vi "SNMP Type to String.vi"(1 "Data":u8[](array[numeric]) format="%.0x", 2 "Type":u8) -> (0 "TypeAsString":string)   [LabVIEW 2017]
doc: "This VI is used to convert the numeric data to a string representation. The input to this VI is the raw byte array containing the data as read from the PDU. The data will be converted according to the specified data type into an ASCII string."
panel:
  out "OctetStringAsBinary":bool
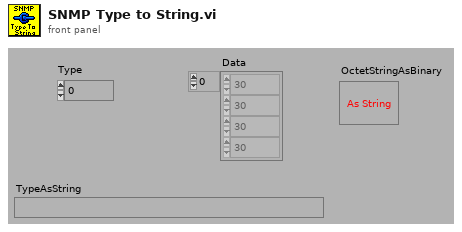
[diagram p1: front panel]
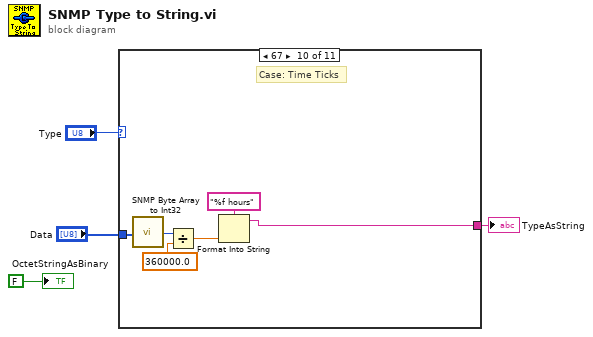
[diagram p0: block diagram]
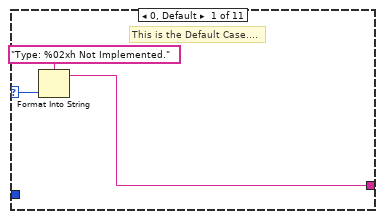
[diagram p2: hidden frame]
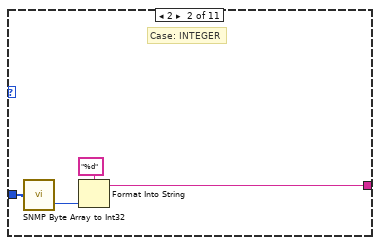
[diagram p3: hidden frame]
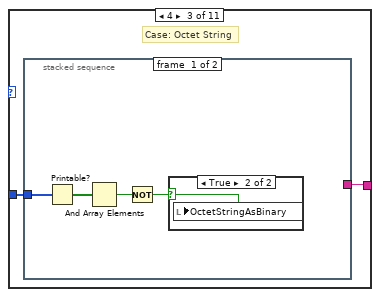
[diagram p4: hidden frame]
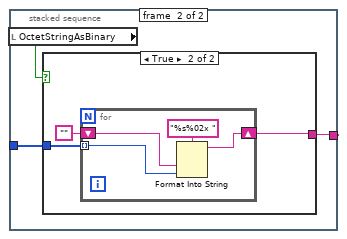
[diagram p6: hidden frame]
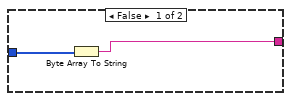
[diagram p7: hidden frame]
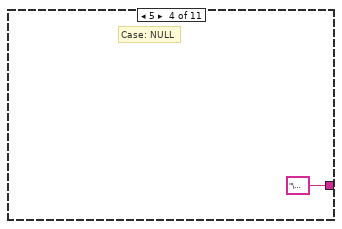
[diagram p8: hidden frame]
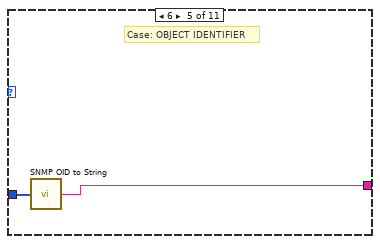
[diagram p9: hidden frame]
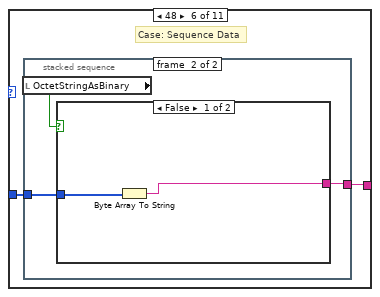
[diagram p10: hidden frame]
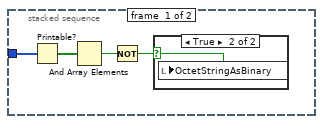
[diagram p11: hidden frame]
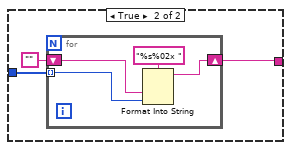
[diagram p13: hidden frame]
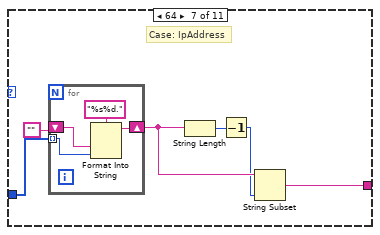
[diagram p14: hidden frame]
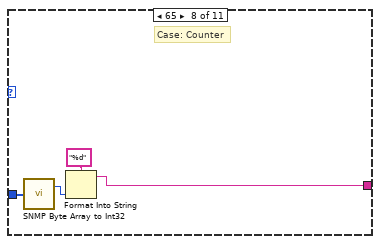
[diagram p15: hidden frame]
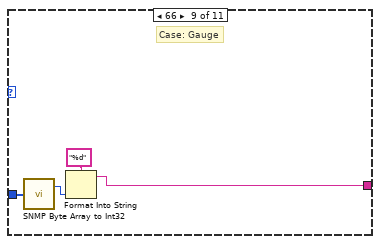
[diagram p16: hidden frame]
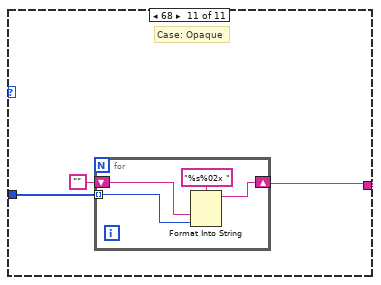
[diagram p17: hidden frame]
diagram:
  n1 = case shown="67" "Type" {
    selector: "Type" -> [w6 _ _ _ _ _ _ _ _ _ _]
    tunnel: "Data" -> [_ w10 w13 _ w33 w35 w57 w65 w68 w72 w79]
    tunnel: [w5 w9 w12 "\u0000" w32 w34 w53 w64 w67 w73 w78] -> w2
    frame 0, Default {
      # "This is the Default Case...."
      n2 = Format Into String(format string="Type: %02xh Not Implemented." ("OID String"), w6) -> (resulting string=w5:string)  [unwired: 2 in, 1 out]
    }
    frame 2 {
      # "Case: INTEGER"
      n3 = call "SNMP Byte Array to Int32.vi"("DataArray"=w10) -> ("Signed Value"=w8:i32)  [unwired: 1 out]
      n4 = Format Into String(format string="%d", w8) -> (resulting string=w9:string)  [unwired: 2 in, 1 out]
    }
    frame 4 {
      # "Case: Octet String"
      n5 = stacked-sequence {
        tunnel: w13 -> [w17 w20]
        tunnel: [_ w19] -> w12
        frame #0 {
          n6 = Printable?(1:w17) -> (0:w16:bool[])
          n7 = And Array Elements(Boolean array=w16) -> (logical AND=w15:bool)
          n8 = Not(x=w15) -> (.not. x?=w14:bool)
          n9 = case shown="True" w14 {
            selector: w14 -> [_ w18]
            frame False {
            }
            frame True {
              n10 = local write "OctetStringAsBinary"(w18) -> ()
            }
          }
        }
        frame #1 {
          n11 = local read "OctetStringAsBinary"() -> (w21:bool)
          n12 = case shown="True" w21 {
            tunnel: w20 -> [w23 w26]
            tunnel: [w22 w25] -> w19
            frame False {
              n13 = Byte Array To String(unsigned byte array=w23) -> (string=w22:string)
            }
            frame True {
              n14 = for {
                tunnel: w26 -> [w29] mode=indexing
                shift-right: [w27] -> w25
                shift-left: "" -> [w28]
                n15 = Format Into String(format string="%s%02x ", w28, w29) -> (resulting string=w27:string)  [unwired: 2 in, 1 out]
              }
            }
          }
        }
      }
    }
    frame 5 {
      # "Case: NULL"
    }
    frame 6 {
      # "Case: OBJECT IDENTIFIER"
      n16 = call "SNMP OID to String.VI"("OID"=w33) -> ("OID String"=w32:string)
    }
    frame 48 {
      # "Case: Sequence Data"
      n17 = stacked-sequence {
        tunnel: w35 -> [w39 w42]
        tunnel: [_ w41] -> w34
        frame #0 {
          n18 = Printable?(1:w39) -> (0:w38:bool[])
          n19 = And Array Elements(Boolean array=w38) -> (logical AND=w37:bool)
          n20 = Not(x=w37) -> (.not. x?=w36:bool)
          n21 = case shown="True" w36 {
            selector: w36 -> [_ w40]
            frame False {
            }
            frame True {
              n22 = local write "OctetStringAsBinary"(w40) -> ()
            }
          }
        }
        frame #1 {
          n23 = local read "OctetStringAsBinary"() -> (w43:bool)
          n24 = case shown="False" w43 {
            tunnel: w42 -> [w45 w48]
            tunnel: [w44 w47] -> w41
            frame False {
              n25 = Byte Array To String(unsigned byte array=w45) -> (string=w44:string)
            }
            frame True {
              n26 = for {
                tunnel: w48 -> [w51] mode=indexing
                shift-right: [w49] -> w47
                shift-left: "" -> [w50]
                n27 = Format Into String(format string="%s%02x ", w50, w51) -> (resulting string=w49:string)  [unwired: 2 in, 1 out]
              }
            }
          }
        }
      }
    }
    frame 64 {
      # "Case: IpAddress"
      n28 = for {
        tunnel: w57 -> [w61] mode=indexing
        shift-right: [w59] -> w56
        shift-left: "" -> [w60]
        n29 = Format Into String(format string="%s%d.", w60, w61) -> (resulting string=w59:string)  [unwired: 2 in, 1 out]
      }
      n30 = String Length(string=w56) -> (length=w55:i32)
      n31 = Decrement(x=w55) -> (x-1=w54:i32)
      n32 = String Subset(string=w56, length (rest)=w54) -> (substring=w53:string)  [unwired: 1 out]
    }
    frame 65 {
      # "Case: Counter"
      n33 = call "SNMP Byte Array to Int32.vi"("DataArray"=w65) -> ("Unsigned Value"=w63:u32)  [unwired: 1 out]
      n34 = Format Into String(format string="%d", w63) -> (resulting string=w64:string)  [unwired: 2 in, 1 out]
    }
    frame 66 {
      # "Case: Gauge"
      n35 = call "SNMP Byte Array to Int32.vi"("DataArray"=w68) -> ("Unsigned Value"=w69:u32)  [unwired: 1 out]
      n36 = Format Into String(format string="%d", w69) -> (resulting string=w67:string)  [unwired: 2 in, 1 out]
    }
    frame 67 {
      # "Case: Time Ticks"
      n37 = call "SNMP Byte Array to Int32.vi"("DataArray"=w72) -> ("Unsigned Value"=w71:u32)  [unwired: 1 out]
      n38 = Divide(x=w71, y=360000.0) -> (x/y=w75:dbl)
      n39 = Format Into String(format string="%f hours", w75) -> (resulting string=w73:string)  [unwired: 2 in, 1 out]
    }
    frame 68 {
      # "Case: Opaque"
      n40 = for {
        tunnel: w79 -> [w82] mode=indexing
        shift-right: [w80] -> w78
        shift-left: "" -> [w81]
        n41 = Format Into String(format string="%s%02x ", w81, w82) -> (resulting string=w80:string)  [unwired: 2 in, 1 out]
      }
    }
  }
  "TypeAsString" <- w2
  "OctetStringAsBinary" <- FALSE ("OctetStringAsBinary")
